vi "Serial Comms - Command and query -simple.vi"(5 "Read response? (T)":bool=TRUE, 7 "Send command? (T)":bool=TRUE, 8 "error in (no error)":errorcluster, 10 "string to write":string="*IDN?\r\n", 11 "Serial Comms in":refnum<class "Serial Comms.lvclass">) -> (0 "error out":errorcluster, 1 "bytes read":u32, 2 "read string":string, 3 "Serial Comms out":refnum<class "Serial Comms.lvclass">, 4 "Empty response string":bool)   [LabVIEW 2020, in "Generic_Comms.lvlib" / "Serial Comms.lvclass"]
uses:
  Serial Comms.lvclass
  Serial Comms.lvclass/Serial Comms.ctl
panel:
  in  "delay after read (ms)":u32=50
  in  "delay before read (ms)":u32=60
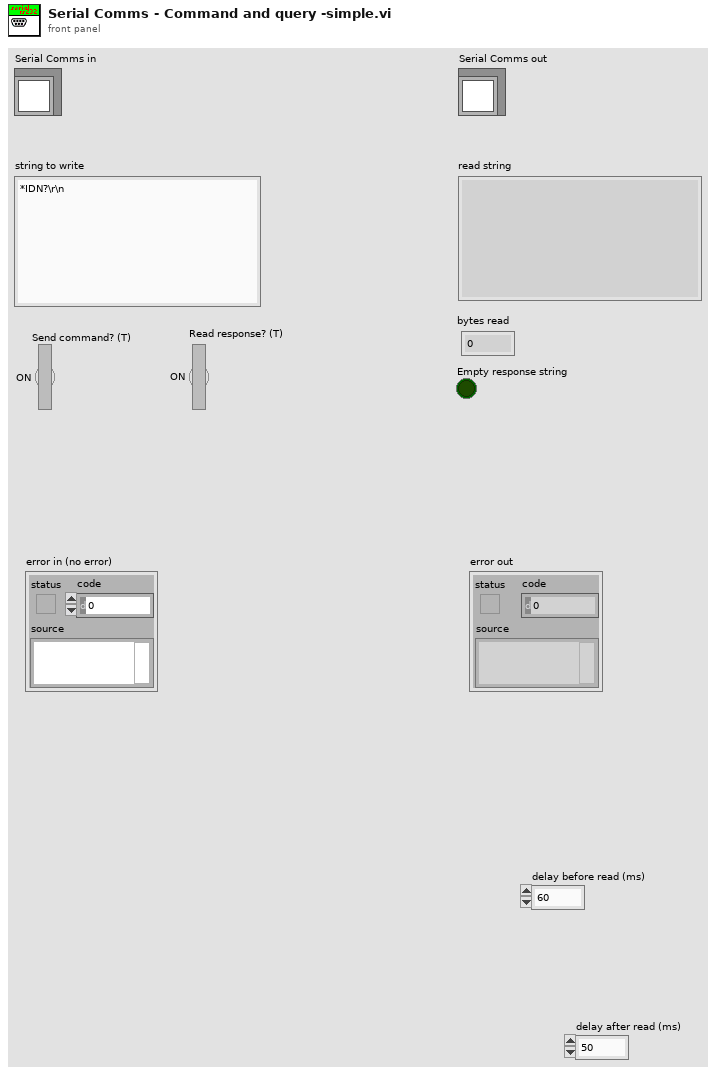
[diagram p1: front panel]
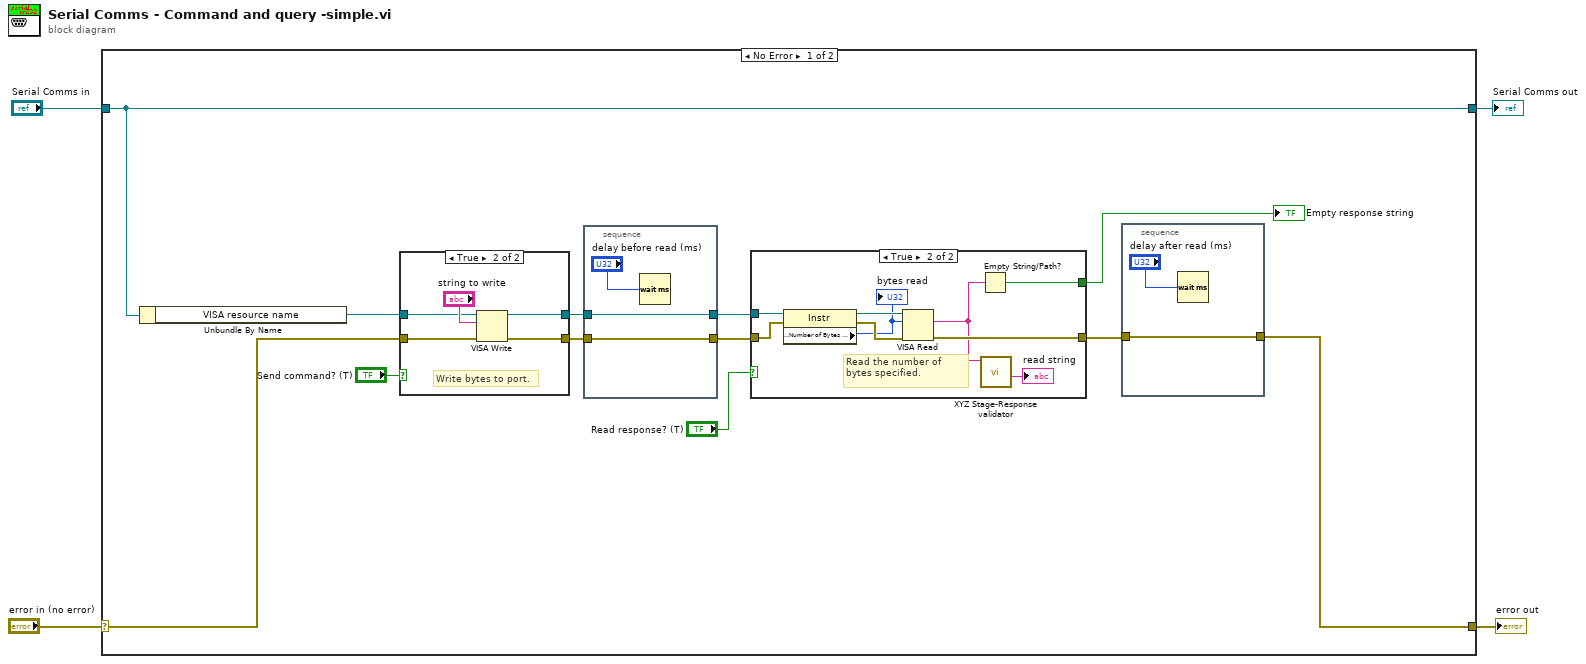
[diagram p0: block diagram]
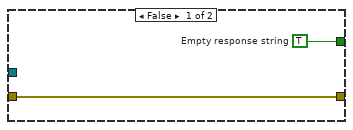
[diagram p2: hidden frame]
diagram:
  n1 = case shown="No Error" "error in (no error)" {
    selector: "error in (no error)" -> [w6 w41]
    tunnel: [w5 w41] -> w3
    tunnel: [w13 w40] -> w1
    tunnel: "Serial Comms in" -> [w13 w40]
    frame No Error {
      n2 = Unbundle By Name(w13) -> ("VISA resource name"=w12:refnum<visa-resource-name>)
      n3 = case shown="True" "Send command? (T)" {
        tunnel: [w34 w39] -> w15
        tunnel: w12 -> [w33 w37]
        tunnel: w6 -> [w34 w36]
        tunnel: [w33 w35] -> w14
        frame False {
        }
        frame True {
          # "Write bytes to port."
          n4 = VISA Write(VISA resource name=w37, write buffer="string to write", error in (no error)=w36) -> (VISA resource name out=w35:refnum<visa-resource-name>, error out=w39:errorcluster)  [unwired: 1 out]
        }
      }
      n5 = stacked-sequence {
        tunnel: w15 -> [w32]
        tunnel: [w32] -> w7
        tunnel: w14 -> [w31]
        tunnel: [w31] -> w8
        frame #0 {
          n6 = Wait (ms)(milliseconds to wait="delay before read (ms)") -> ()  [unwired: 1 out]
        }
      }
      n7 = case shown="True" "Read response? (T)" {
        tunnel: w7 -> [w20 w26]
        tunnel: [w20 w29] -> w10
        tunnel: w8 -> [_ w28]
        tunnel: [w19 w23] -> w9
        frame False {
          w19 = TRUE  # Empty response string
        }
        frame True {
          # "Read the number of bytes specified."
          n8 = property class="Instr"(reference=w28, error in=w26) -> (reference out=w27:refnum<visa-resource-name>, error out=w25:errorcluster, "Serial Settings:Number of Bytes at Serial Port"=w24:u32)
          "bytes read" <- w24
          n9 = VISA Read(VISA resource name=w27, byte count=w24, error in (no error)=w25) -> (read buffer=w22:string, error out=w29:errorcluster)  [unwired: 2 out]
          n10 = Empty String/Path?(string/path=w22) -> (empty?=w23:bool)
          n11 = call "XYZ Stage-Response validator.vi"("response string"=w22) -> ("Filtered response"=→"read string":string)  [unwired: 9 in, 1 out]
        }
      }
      "Empty response string" <- w9
      n12 = stacked-sequence {
        tunnel: w10 -> [w18]
        tunnel: [w18] -> w5
        frame #0 {
          n13 = Wait (ms)(milliseconds to wait="delay after read (ms)") -> ()  [unwired: 1 out]
        }
      }
    }
    frame Error {
    }
  }
  "error out" <- w3
  "Serial Comms out" <- w1
